vi "EditorThumbnail mouseRelease.vi"(8 "error in (no error)":errorcluster, 11 "EditorThumbnail in":refnum<class "EditorThumbnail.lvclass">) -> (0 "error out":errorcluster, 3 "EditorThumbnail out":refnum<class "EditorThumbnail.lvclass">)   [LabVIEW 2018, in "EditorThumbnail.lvclass"]
uses:
  EditorThumbnail.lvclass
  EditorThumbnail.lvclass/EditorThumbnail.ctl
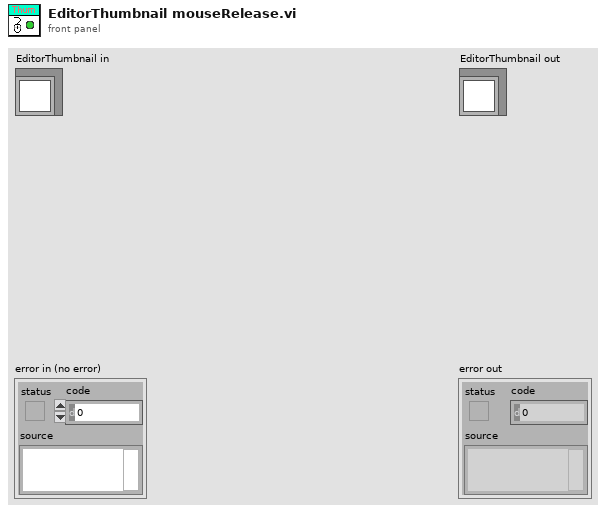
[diagram p1: front panel]
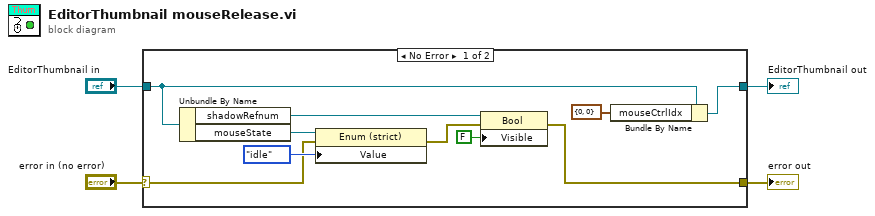
[diagram p0: block diagram]
diagram:
  n1 = case shown="No Error" "error in (no error)" {
    selector: "error in (no error)" -> [w12 w16]
    tunnel: [w5 w16] -> w3
    tunnel: [w9 w15] -> w1
    tunnel: "EditorThumbnail in" -> [w11 w15]
    frame No Error {
      n2 = Unbundle By Name(w11) -> ("shadowRefnum"=w7:refnum<vi>, "mouseState"=w14:refnum<vi>)
      n3 = property class="Enum (strict)"(reference=w14, error in=w12, "Value"=enum16{"idle", "down", "move", "up"}."idle") -> (error out=w6:errorcluster)  [unwired: 1 out]
      n4 = property class="Bool"(reference=w7, error in=w6, "Visible"=FALSE) -> (error out=w5:errorcluster)  [unwired: 1 out]
      n5 = Bundle By Name(cluster=w11, "mouseCtrlIdx"=cluster{"downIdx":i32, "upIdx":i32} {"downIdx"=0, "upIdx"=0}) -> (w9:refnum<class "EditorThumbnail.lvclass">)
    }
    frame Error {
    }
  }
  "error out" <- w3
  "EditorThumbnail out" <- w1
